vi "Ctor.vi"(8 "error in (no error)":errorcluster, 11 "Update Event":refnum<user-event>) -> (0 "error out":errorcluster, 3 "Blueprint out":refnum<class "Blueprint.lvclass">)   [LabVIEW 2020, in "Blueprint.lvclass"]
uses:
  Blueprint.lvclass
  Ref Data.ctl
  Item/Ingredient.ctl
  Item/Item.lvclass
  Workstation/Workstation.lvclass
  Blueprint.lvclass/Blueprint.ctl
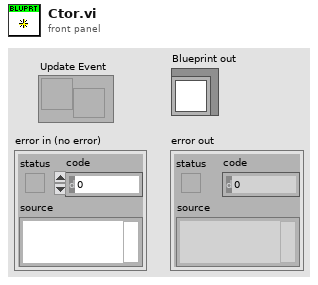
[diagram p1: front panel]
types:
  T1 = typedef "Blueprint.lvclass/Ref Data.ctl" = cluster{"Ingredients":T2[], "Workstation":refnum<class "Workstation.lvclass">, "Craft Time":dbl, "Name":string}
  T2 = typedef "Item.lvclass/Ingredient.ctl" = cluster{"Item":refnum<class "Item.lvclass">, "Qty":dbl}
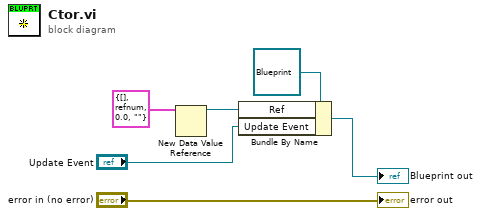
[diagram p0: block diagram]
diagram:
  n1 = New Data Value Reference(data value=T1 {"Ingredients"=[], "Workstation"=refnum, "Craft Time"=0.0, "Name"=""} ("Ref Data")) -> (data value reference=w2:refnum<data-value>)  [unwired: 1 in, 1 out]
  n2 = Bundle By Name(cluster=refnum<class "Blueprint.lvclass"> refnum ("Blueprint in"), "Ref"=w2, "Update Event"="Update Event") -> (→"Blueprint out":refnum<class "Blueprint.lvclass">)
  "error out" <- "error in (no error)"
